vi "get_config_cluster.vi"(8 "error in (no error)":errorcluster, 11 "ScanHeadMH100729FPGA in":refnum<class "ScanHeadMH100729FPGA.lvclass">) -> (0 "error out":errorcluster, 2 "config cluster (variant)":variant, 3 "ScanHeadMH100729FPGA out":refnum<class "ScanHeadMH100729FPGA.lvclass">)   [LabVIEW 2010, in "ScanHeadMH100729FPGA.lvclass"]
uses:
  ScanHeadMH100729FPGA.lvclass
  ScanHeadMH100729FPGA.lvclass/ScanHeadMH100729FPGA.ctl
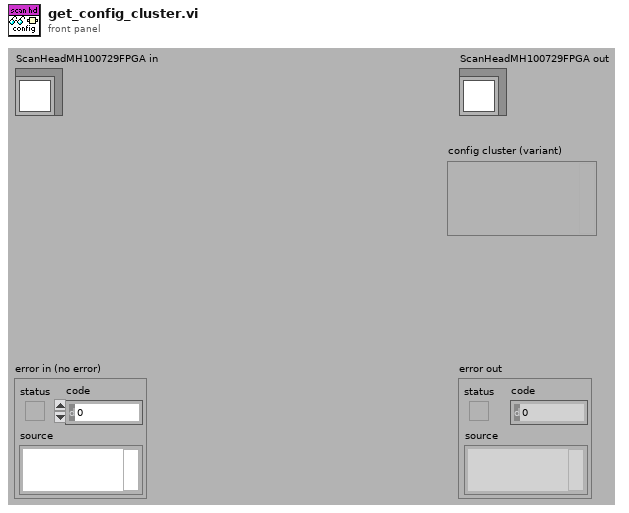
[diagram p1: front panel]
types:
  T1 = typedef "ScanHeadMH100729FPGA.lvclass/config_data_cluster.ctl" = cluster{"visibility":cluster{"Zoom":bool, "RotateX":bool, "RotateY":bool, "TranslateX":bool, "TranslateY":bool, "TranslateZ":bool}, "subcomponent specifications":cluster{"intensity modifier":T2}, "translation factor":dbl[unit]}
  T2 = typedef "plugin_specification.ctl" = cluster{"class path":string, "configuration":string, "label":string, "settings name":string}
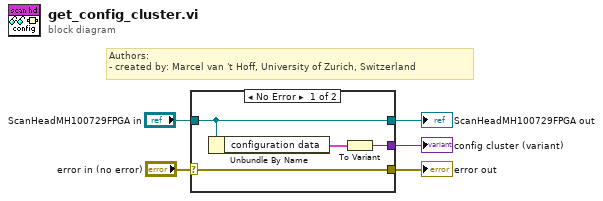
[diagram p0: block diagram]
diagram:
  # "Authors: \n- created by: Marcel van 't Hoff, University of Zurich, Switzerland"
  n1 = case shown="No Error" "error in (no error)" {
    selector: "error in (no error)" -> [w9 w11]
    tunnel: [w9 w11] -> w4
    tunnel: [w8 w10] -> w3
    tunnel: "ScanHeadMH100729FPGA in" -> [w8 w10]
    tunnel: [w6 _] -> w1
    frame No Error {
      n2 = Unbundle By Name(w8) -> ("configuration data"=w7:T1)
      n3 = To Variant(anything=w7) -> (Variant=w6:variant)
    }
    frame Error {
    }
  }
  "error out" <- w4
  "ScanHeadMH100729FPGA out" <- w3
  "config cluster (variant)" <- w1
